vi "ASI_READxyz.vi"(8 "error in (no error)":errorcluster, 11 "VISA resource name":refnum<visa-resource-name>) -> (0 "error out":errorcluster, 1 "y [mm]":dbl, 2 "x [mm]":dbl, 3 "VISA resource name out":refnum<visa-resource-name>, 5 "z [mm]":dbl)   [LabVIEW 2011]
uses:
  <vilib>/Instr/_visa.llb/VISA Flush IO Buffer Mask.ctl
panel:
  out "read buffer":string
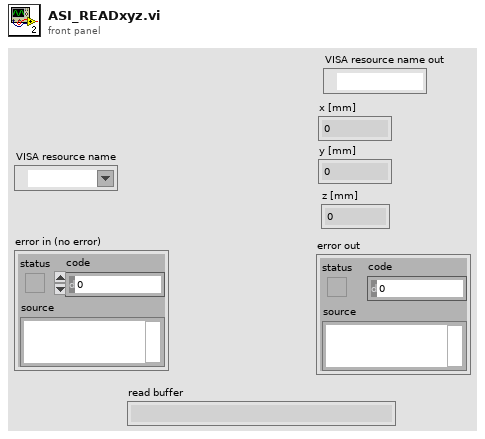
[diagram p1: front panel]
types:
  T1 = typedef "VISA Flush IO Buffer Mask.ctl" = u16
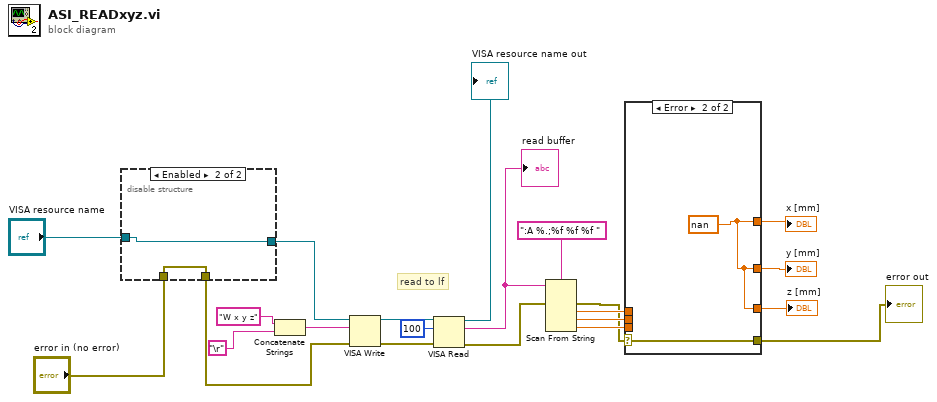
[diagram p0: block diagram]
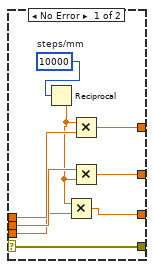
[diagram p2: hidden frame]
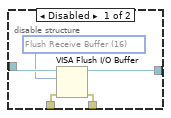
[diagram p3: hidden frame]
diagram:
  # "read to lf"
  n1 = disable-structure shown="Enabled" {
    disable-tunnel: "VISA resource name" -> [w27 w29]
    disable-tunnel: [w26 w29] -> w15
    disable-tunnel: "error in (no error)" -> [w24 w28]
    disable-tunnel: [w23 w28] -> w13
    frame Disabled {
      w25 = T1 16 items=["Flush Receive Buffer"=16, "Write Transmit Buffer to Device"=32, "Flush Receive Buffer (No I/O)"=64, "Flush Transmit Buffer"=128] ("Mask")
      n2 = VISA Flush I/O Buffer(VISA resource name=w27, mask (16)=w25, error in (no error)=w24) -> (VISA resource name out=w26:refnum<visa-resource-name>, error out=w23:errorcluster)
    }
    frame Enabled {
    }
  }
  n3 = Concatenate Strings("W x y z" ("write buffer"), "\r") -> (w20:string)
  n4 = VISA Write(VISA resource name=w15, write buffer=w20, error in (no error)=w13) -> (VISA resource name out=w18:refnum<visa-resource-name>, error out=w16:errorcluster)  [unwired: 1 out]
  n5 = VISA Read(VISA resource name=w18, byte count=u32 100, error in (no error)=w16) -> (VISA resource name out=→"VISA resource name out":refnum<visa-resource-name>, read buffer=w12:string, error out=w7:errorcluster)  [unwired: 1 out]
  "read buffer" <- w12
  n6 = Scan From String(format string=":A %.;%f %f %f ", input string=w12, error in=w7) -> (error out=w5:errorcluster, output 1=w10:dbl, output 2=w9:dbl, output 3=w8:dbl)  [unwired: 4 in, 2 out]
  n7 = case shown="Error" w5 {
    selector: w5 -> [w33 w40]
    tunnel: w10 -> [w38 _]
    tunnel: w9 -> [w37 _]
    tunnel: w8 -> [w36 _]
    tunnel: [w33 w40] -> w4
    tunnel: [w32 w39] -> w3
    tunnel: [w31 w39] -> w2
    tunnel: [w30 w39] -> w1
    frame No Error {
      w35 = 10000  # steps/mm
      n8 = Reciprocal(x=w35) -> (1/x=w34:dbl)
      n9 = Multiply(x=w34, y=w36) -> (x*y=w30:dbl)
      n10 = Multiply(x=w34, y=w38) -> (x*y=w32:dbl)
      n11 = Multiply(x=w37, y=w34) -> (x*y=w31:dbl)
    }
    frame Error {
      w39 = nan
    }
  }
  "error out" <- w4
  "x [mm]" <- w3
  "y [mm]" <- w2
  "z [mm]" <- w1
